vi "InitScan.vi"(8 "error in (no error)":errorcluster, 10 "Total Steps":u16, 11 "Spectroscopy_Controller in":refnum<class "Spectroscopy_Controller.lvclass">) -> (0 "error out":errorcluster, 3 "Spectroscopy_Controller out":refnum<class "Spectroscopy_Controller.lvclass">)   [LabVIEW 2023, in "Spectroscopy_Controller.lvlib" / "Spectroscopy_Controller.lvclass"]
uses:
  Spectroscopy_Controller.lvclass
  UIs/Camera_Controller/Camera_Controller Messages/External_Acq Msg/External_Acq Msg.lvclass
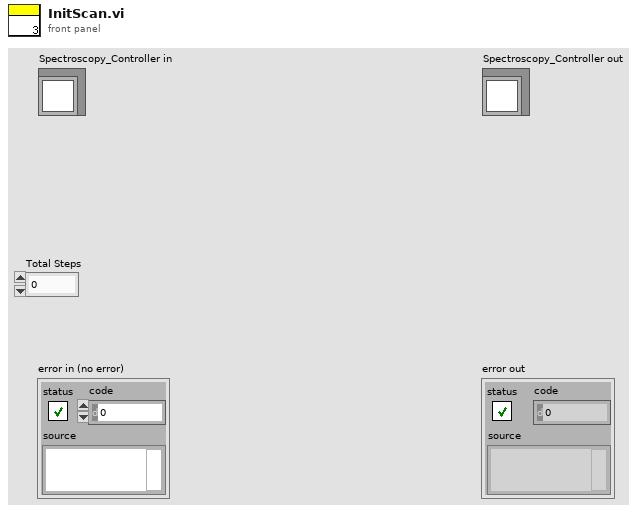
[diagram p1: front panel]
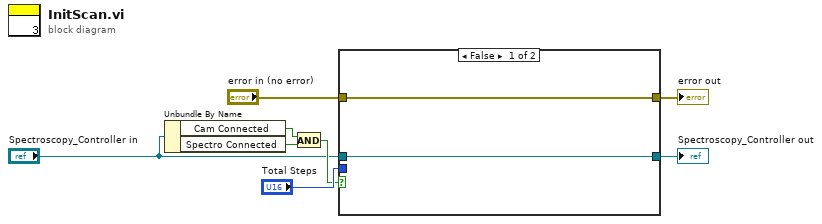
[diagram p0: block diagram]
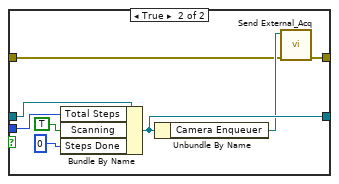
[diagram p2: hidden frame]
diagram:
  n1 = Unbundle By Name("Spectroscopy_Controller in") -> ("Cam Connected"=w7:bool, "Spectro Connected"=w6:bool)
  n2 = And(x=w7, y=w6) -> (x .and. y?=w5:bool)
  n3 = case shown="False" w5 {
    tunnel: [w9 w13] -> w2
    tunnel: [w10 w15] -> w1
    tunnel: "Spectroscopy_Controller in" -> [w10 w18]
    tunnel: "Total Steps" -> [_ w12]
    tunnel: "error in (no error)" -> [w9 w11]
    frame False {
    }
    frame True {
      n4 = Bundle By Name(cluster=w18, "Total Steps"=w12, "Scanning"=TRUE, "Steps Done"=u16 0) -> (w15:refnum<class "Spectroscopy_Controller.lvclass">)
      n5 = Unbundle By Name(w15) -> ("Camera Enqueuer"=w14:refnum<class "Message Enqueuer.lvclass">)
      n6 = call "Send External_Acq.vi"("error in (no error)"=w11, "Message Enqueuer"=w14) -> ("error out"=w13:errorcluster)  [unwired: 8 in, 1 out]
    }
  }
  "error out" <- w2
  "Spectroscopy_Controller out" <- w1
